vi "readInWave.vi"() -> ()   [LabVIEW 2011, in "run.lvlib"]
uses:
  run.lvlib
panel:
  out "Data":dbl[](array[numeric])
  in  "channel":string
  out "timeLength":dbl
  in  "Path":path
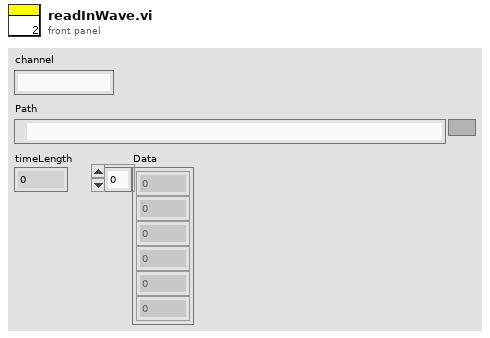
[diagram p1: front panel]
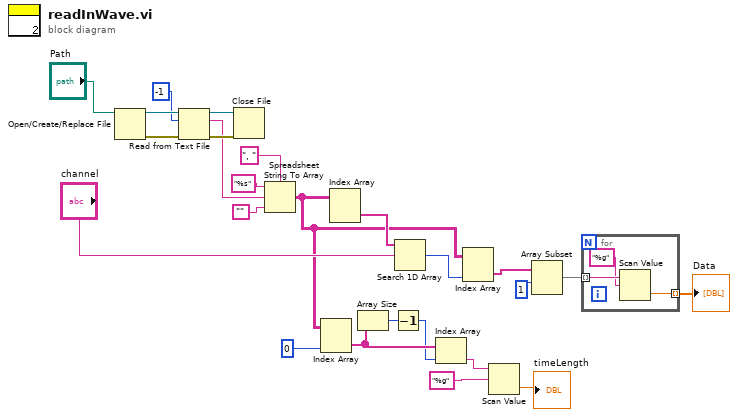
[diagram p0: block diagram]
diagram:
  n1 = Open/Create/Replace File(file path (use dialog)="Path") -> (refnum out=w25:refnum<file>, error out=w24:errorcluster)  [unwired: 5 in, 1 out]
  n2 = Read from Text File(file (use dialog)=w25, count=-1, error in=w24) -> (refnum out=w22:refnum<file>, text=w19:string, error out=w23:errorcluster)  [unwired: 1 in, 1 out]
  n3 = Close File(refnum=w22, error in=w23) -> ()  [unwired: 2 out]
  n4 = Spreadsheet String To Array(delimiter (Tab)=", ", format string="%s", spreadsheet string=w19, array type (2D Dbl)="") -> (array=w8:string[][])
  n5 = Index Array(array=w8, index (col)=0 ("disabled index (col)")) -> (element=w5:string[])  [unwired: 1 in]
  n6 = Index Array(array=w8) -> (element=w15:string[])  [unwired: 2 in]
  n7 = Array Size(array=w5) -> (size(s)=w4:i32)
  n8 = Decrement(x=w4) -> (x-1=w1:i32)
  n9 = Search 1D Array(1D array=w15, element="channel") -> (index of element=w13:i32)  [unwired: 1 in]
  n10 = Index Array(array=w5, index=w1) -> (element=w3:string)
  n11 = Index Array(array=w8, index (col)=w13) -> (element=w12:string[])  [unwired: 1 in]
  n12 = Scan Value(string=w3, format string="%g") -> (value=→"timeLength":dbl)  [unwired: 1 in, 1 out]
  n13 = Array Subset(array=w12, index=1) -> (w10:string[])  [unwired: 1 in]
  n14 = for {
    tunnel: w10 -> [w28] mode=indexing
    tunnel: [w26] -> w9 mode=indexing
    n15 = Scan Value(string=w28, format string="%g") -> (value=w26:dbl)  [unwired: 1 in, 1 out]
  }
  "Data" <- w9
